vi "bank.vi"() -> ()   [LabVIEW 2018]
panel:
  in  "Withdraw":bool
  in  "Deposit":bool
  out "Balance":dbl
  in  "Amount":dbl
  in  "stop":bool
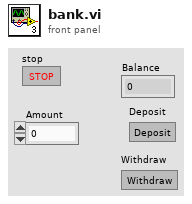
[diagram p1: front panel]
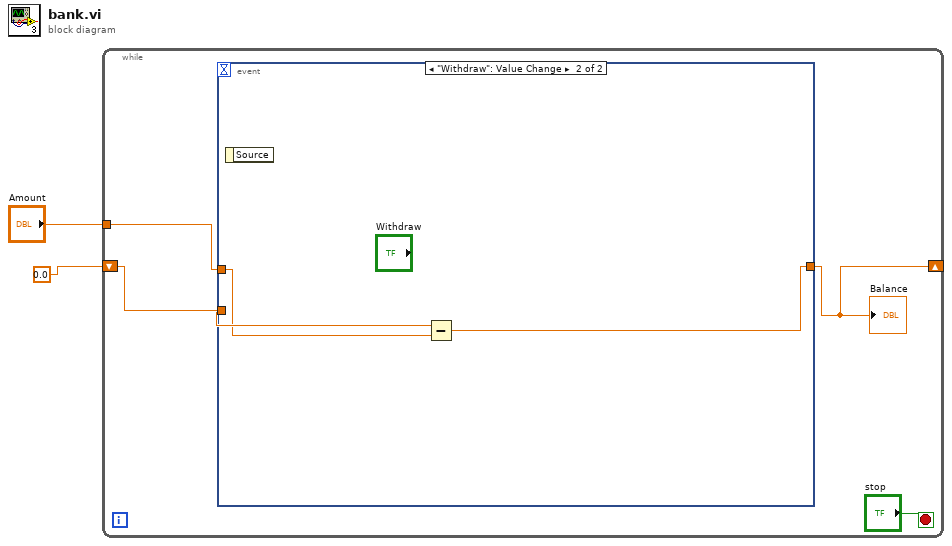
[diagram p0: block diagram]
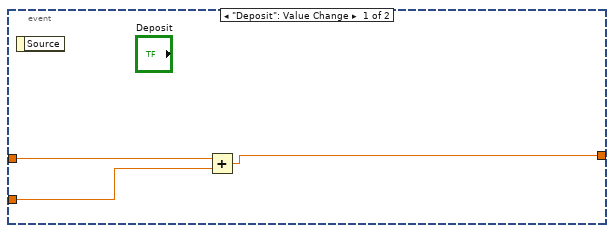
[diagram p2: hidden frame]
diagram:
  n1 = while {
    shift-right: [w3] -> _
    shift-left: 0.0 -> [w5]
    tunnel: "Amount" -> [w4]
    stop <- "stop" stop-if-true
    n2 = event shown="[1] \"Withdraw\": Value Change" {
      selector: _ -> [_ _]
      dyn-events: _ -> [_ _]
      timeout: _ -> [_ _]
      tunnel: w5 -> [w9 w12]
      tunnel: [w8 w11] -> w3
      tunnel: w4 -> [w7 w10]
      event "Deposit": Value Change {
        n3 = event-data() -> ()  [unwired: 1 in, 1 out]
        n4 = Add(x=w7, y=w9) -> (x+y=w8:dbl)
      }
      event "Withdraw": Value Change {
        n5 = event-data() -> ()  [unwired: 1 in, 1 out]
        n6 = Subtract(x=w12, y=w10) -> (x-y=w11:dbl)
      }
    }
    "Balance" <- w3
  }
